vi "Inst.RP100.getAll.vi"(8 "error in (no error)":errorcluster, 11 "Inst.RP100 in":refnum<class "Inst.RP100.lvclass">) -> (0 "error out":errorcluster, 2 "output cluster":T1, 3 "Inst.RP100 out":refnum<class "Inst.RP100.lvclass">)   [LabVIEW 2019, in "Inst.RP100.lvclass"]
uses:
  Inst.RP100.lvclass
  Typedefs/Inst.RP100.getAll--Cluster.ctl
  Typedefs/Output Channel--Enum.ctl
  Inst.RP100.lvclass/Inst.RP100.ctl
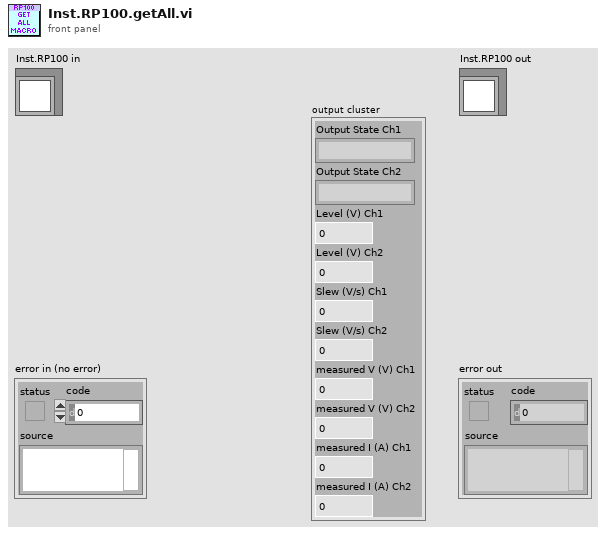
[diagram p1: front panel]
types:
  T1 = typedef "Inst.RP100.lvclass/Inst.RP100.getAll--Cluster.ctl" = cluster{"Output State Ch1":string, "Output State Ch2":string, "Level (V) Ch1":dbl, "Level (V) Ch2":dbl, "Slew (V/s) Ch1":dbl, "Slew (V/s) Ch2":dbl, "measured V (V) Ch1":dbl, "measured V (V) Ch2":dbl, "measured I (A) Ch1":dbl, "measured I (A) Ch2":dbl}
  T2 = typedef "Inst.RP100.lvclass/Output Channel--Enum.ctl" = enum16{"Output 1", "Output 2"}
  T3 = typedef "Inst.RP100.lvclass/Output State--Enum.ctl" = enum16{"Shorted", "Enabled"}
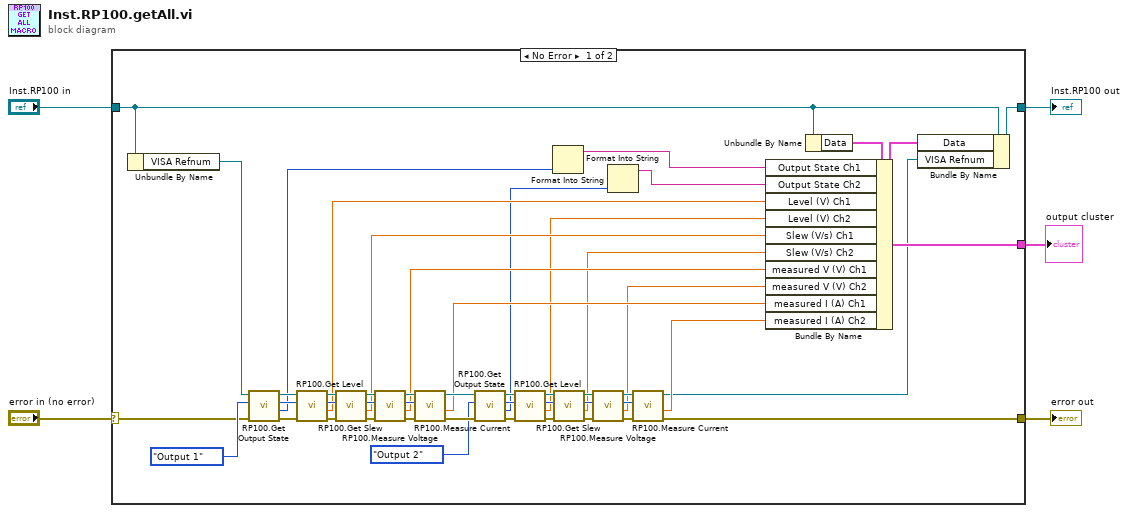
[diagram p0: block diagram]
diagram:
  n1 = case shown="No Error" "error in (no error)" {
    selector: "error in (no error)" -> [w8 w55]
    tunnel: [w11 w55] -> w3
    tunnel: [w16 w54] -> w2
    tunnel: "Inst.RP100 in" -> [w10 w54]
    tunnel: [w7 _] -> w1
    frame No Error {
      n2 = Unbundle By Name(w10) -> ("VISA Refnum"=w9:refnum<visa-resource-name>)
      n3 = call "RP100.Get Output State.vi"("error in (no error)"=w8, "Output Channel"=Output_Channel--Enum."Output 1", "VISA resource name"=w9) -> ("error out"=w42:errorcluster, "Output State"=w15:T3, "Output Channel"=w31:T2, "VISA Refnum out"=w43:refnum<visa-resource-name>)  [unwired: 5 in]
      n4 = call "RP100.Get Level.vi"("error in (no error)"=w42, "Output Channel"=w31, "VISA resource name"=w43) -> ("error out"=w40:errorcluster, "Level (V)"=w25:dbl, "Output Channel"=w30:T2, "VISA Refnum out"=w41:refnum<visa-resource-name>)  [unwired: 5 in]
      n5 = call "RP100.Get Slew.vi"("error in (no error)"=w40, "Output Channel"=w30, "VISA resource name"=w41) -> ("error out"=w38:errorcluster, "Slew (V/s)"=w24:dbl, "Output Channel"=w29:T2, "VISA Refnum out"=w39:refnum<visa-resource-name>)  [unwired: 5 in]
      n6 = call "RP100.Measure Voltage.vi"("error in (no error)"=w38, "Output"=w29, "VISA resource name"=w39) -> ("error out"=w52:errorcluster, "measured V"=w23:dbl, "Output"=w51:T2, "VISA Refnum out"=w53:refnum<visa-resource-name>)  [unwired: 5 in]
      n7 = call "RP100.Measure Current.vi"("error in (no error)"=w52, "Output Channel"=w51, "VISA resource name"=w53) -> ("error out"=w47:errorcluster, "measured I"=w22:dbl, "VISA Refnum out"=w46:refnum<visa-resource-name>)  [unwired: 5 in, 1 out]
      n8 = call "RP100.Get Output State.vi"("error in (no error)"=w47, "Output Channel"=Output_Channel--Enum."Output 2", "VISA resource name"=w46) -> ("error out"=w36:errorcluster, "Output State"=w13:T3, "Output Channel"=w28:T2, "VISA Refnum out"=w37:refnum<visa-resource-name>)  [unwired: 5 in]
      n9 = call "RP100.Get Level.vi"("error in (no error)"=w36, "Output Channel"=w28, "VISA resource name"=w37) -> ("error out"=w34:errorcluster, "Level (V)"=w21:dbl, "Output Channel"=w27:T2, "VISA Refnum out"=w35:refnum<visa-resource-name>)  [unwired: 5 in]
      n10 = Format Into String(w15) -> (resulting string=w14:string)  [unwired: 3 in, 1 out]
      n11 = call "RP100.Get Slew.vi"("error in (no error)"=w34, "Output Channel"=w27, "VISA resource name"=w35) -> ("error out"=w32:errorcluster, "Slew (V/s)"=w20:dbl, "Output Channel"=w26:T2, "VISA Refnum out"=w33:refnum<visa-resource-name>)  [unwired: 5 in]
      n12 = call "RP100.Measure Voltage.vi"("error in (no error)"=w32, "Output"=w26, "VISA resource name"=w33) -> ("error out"=w49:errorcluster, "measured V"=w19:dbl, "Output"=w50:T2, "VISA Refnum out"=w48:refnum<visa-resource-name>)  [unwired: 5 in]
      n13 = Format Into String(w13) -> (resulting string=w12:string)  [unwired: 3 in, 1 out]
      n14 = call "RP100.Measure Current.vi"("error in (no error)"=w49, "Output Channel"=w50, "VISA resource name"=w48) -> ("error out"=w11:errorcluster, "measured I"=w18:dbl, "VISA Refnum out"=w6:refnum<visa-resource-name>)  [unwired: 5 in, 1 out]
      n15 = Unbundle By Name(w10) -> ("Data"=w17:T1)
      n16 = Bundle By Name(cluster=w17, "Output State Ch1"=w14, "Output State Ch2"=w12, "Level (V) Ch1"=w25, "Level (V) Ch2"=w21, "Slew (V/s) Ch1"=w24, "Slew (V/s) Ch2"=w20, "measured V (V) Ch1"=w23, "measured V (V) Ch2"=w19, "measured I (A) Ch1"=w22, "measured I (A) Ch2"=w18) -> (w7:T1)
      n17 = Bundle By Name(cluster=w10, "Data"=w7, "VISA Refnum"=w6) -> (w16:refnum<class "Inst.RP100.lvclass">)
    }
    frame Error {
    }
  }
  "error out" <- w3
  "Inst.RP100 out" <- w2
  "output cluster" <- w1
